vi "Fire StopProcess Event.vi"(6 "timeout in ms (5000)":i32=5000, 8 "error in (no error)":errorcluster, 11 "Event in":refnum<user-event>) -> (0 "error out":errorcluster, 1 "timed out?":bool, 2 "sync from process?":bool, 3 "Event out":refnum<user-event>)   [LabVIEW 2017]
doc: "Developed by Kevin Thompson\nkevin@thompsonengineering.net\n\nCopyright 2018-2020\nThompson Engineering, LLC\n\n\nVI Shots Reuse Library 2.0.2.27\nCode developed by Michael Aivaliotis - VI Shots"
uses:
  <vilib>/event_ctls.llb/usereventprio.ctl
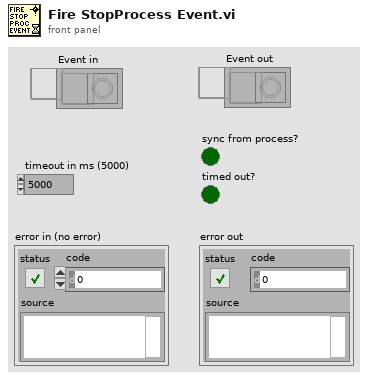
[diagram p1: front panel]
types:
  T1 = typedef "usereventprio.ctl" = enum32{"high priority", "normal priority"}
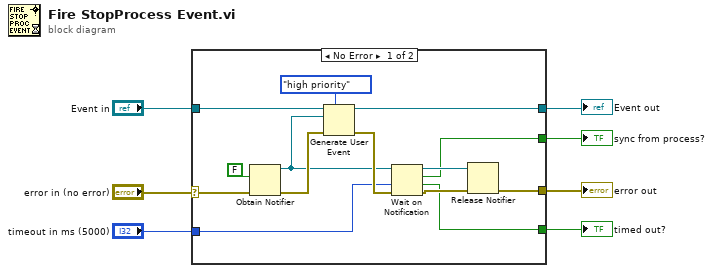
[diagram p0: block diagram]
diagram:
  n1 = case shown="No Error" "error in (no error)" {
    selector: "error in (no error)" -> [w8 w22]
    tunnel: [w21 w22] -> w7
    tunnel: "Event in" -> [w20 w23]
    tunnel: "timeout in ms (5000)" -> [w15 _]
    tunnel: [w11 w23] -> w4
    tunnel: [w10 _] -> w3
    tunnel: [w9 _] -> w2
    frame No Error {
      n2 = Obtain Notifier(notification data type=FALSE, error in (no error)=w8) -> (notifier out=w16:refnum<notifier>, error out=w18:errorcluster)  [unwired: 2 in, 1 out]
      n3 = Generate User Event(priority (normal)=usereventprio."high priority", user event=w20, event data cluster=w16, error in=w18) -> (user event out=w11:refnum<user-event>, error out=w17:errorcluster)
      n4 = Wait on Notification(notifier=w16, timeout in ms (-1)=w15, error in (no error)=w17) -> (notifier out=w14:refnum<notifier>, notification=w10:bool, timed out?=w9:bool, error out=w13:errorcluster)  [unwired: 1 in]
      n5 = Release Notifier(notifier=w14, error in (no error)=w13) -> (error out=w21:errorcluster)  [unwired: 1 in, 2 out]
    }
    frame Error {
    }
  }
  "error out" <- w7
  "Event out" <- w4
  "sync from process?" <- w3
  "timed out?" <- w2
